vi "dll_path.vi"() -> ()   [LabVIEW 2019, in "Haptic Prog Interface.lvlib"]
uses:
  Haptic Prog Interface.lvlib
panel:
  in  "Path":path=path "C:/Users/freem/Documents/GitHub/HapticSPM/Haptic-Programming-Interface/x64/Debug/Haptic Programming Interface.dll"
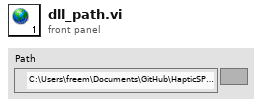
[diagram p1: front panel]
diagram:
